vi "Find_camera.vi"(0 "error in":errorcluster) -> (4 "attribs":variant, 5 "port":u16, 6 "error out":errorcluster, 7 "name":string, 8 "CameraInfo":T1 {"serial" format="%x"}, 9 "CameraBase out":refnum<class "CameraBase.lvclass">)   [LabVIEW 2010]
uses:
  <userlib>/Imaging/classes/CameraBase/CameraBase.lvclass
  <userlib>/Imaging/classes/CameraBase/CameraInfo.ctl
  <userlib>/Imaging/classes/sdk_list.ctl
  <userlib>/Imaging/classes/IMAQdx/IMAQdx.lvclass
  <userlib>/Imaging/classes/AndorSDK2/AndorSDK2.lvclass
  <userlib>/h5labview/H5File.lvlib
  <userlib>/h5labview/H5Attrib.lvlib
panel:
  out "h5":path
  in  "cancel":bool
  in  "ok":bool
  in  "cameras":i32(listbox)
  # "Select camera to connect to:"
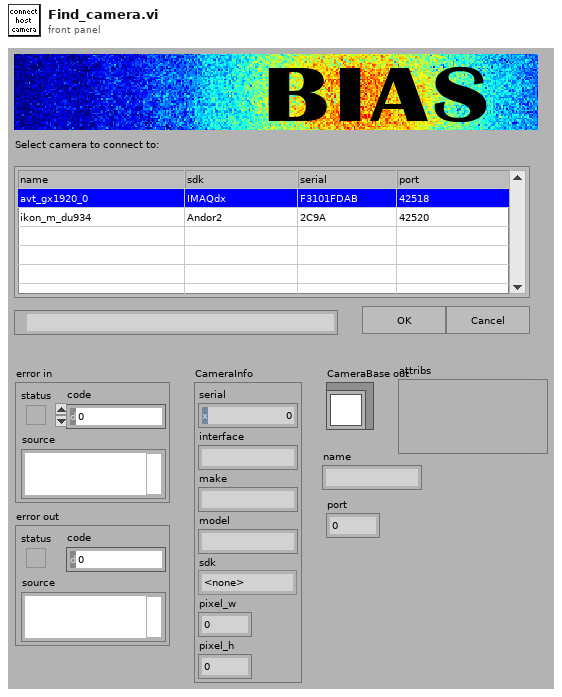
[diagram p1: front panel]
types:
  T1 = typedef "CameraInfo.ctl" = cluster{"serial":u64, "interface":string, "make":string, "model":string, "sdk":T2, "pixel_w":dbl, "pixel_h":dbl}
  T2 = typedef "sdk_list.ctl" = enum16{"<none>", "NIvision", "Andor2", "Andor3"}
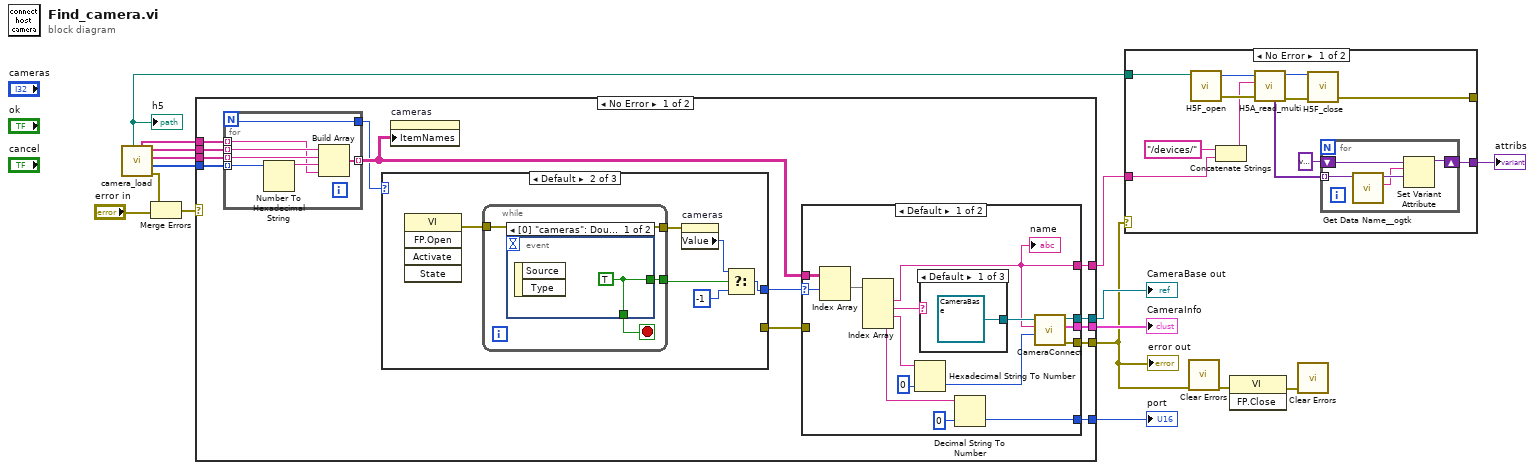
[diagram p0: block diagram]
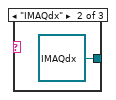
[diagram p3: hidden frame]
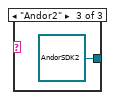
[diagram p4: hidden frame]
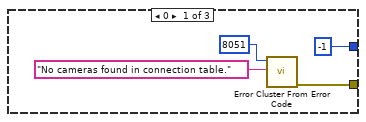
[diagram p6: hidden frame]
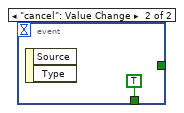
[diagram p7: hidden frame]
diagram:
  n1 = call <userlib>:"camera_load.vi"() -> ("error out"=w14:errorcluster, "serials"=w11:u64[], "sdks"=w10:string[], "names"=w9:string[], "ports"=w8:string[], "hdf"=w5:path)  [unwired: 4 in]
  "h5" <- w5
  n2 = Merge Errors(w14, "error in") -> (w12:errorcluster)
  n3 = case shown="No Error" w12 {
    selector: w12 -> [_ w71]
    tunnel: [w27 w71] -> w2
    tunnel: [w26 _] -> w16
    tunnel: [w25 _] -> w15
    tunnel: w11 -> [w24 _]
    tunnel: w10 -> [w23 _]
    tunnel: w9 -> [w22 _]
    tunnel: w8 -> [w21 _]
    tunnel: [w19 _] -> w7
    tunnel: [w17 _] -> w4
    frame No Error {
      n4 = for {
        N -> [w30]
        tunnel: w22 -> [w36] mode=indexing
        tunnel: w23 -> [w35] mode=indexing
        tunnel: w24 -> [w34] mode=indexing
        tunnel: [w32] -> w20 mode=indexing
        tunnel: w21 -> [w31] mode=indexing
        tunnel: [w30] -> w18
        n5 = Number To Hexadecimal String(2:w34) -> (0:w33:string)  [unwired: 1 in]
        n6 = Build Array(w36, w35, w33, w31) -> (w32:string[])
      }
      n7 = case shown="Default" w18 {
        tunnel: [w58 _ _] -> w28
        tunnel: [-1 ("Value") w61 _] -> w29
        frame 0 {
          n8 = call <vilib>:"Error Cluster From Error Code.vi"("error message (\"\")"="No cameras found in connection table." ("format string"), "error code (0)"=8051) -> ("error out"=w58:errorcluster)  [unwired: 7 in]
        }
        frame Default {
          n9 = invoke class="VI" method="FP.Open"() -> (error out=w60:errorcluster)  [unwired: 5 in, 4 out]
          n10 = while {
            tunnel: w60 -> [w67]
            tunnel: [w68] -> w63
            tunnel: [w67] -> w65
            stop <- w66 stop-if-true
            n11 = event shown="[0] \"cameras\": Double Click;  \"ok\": Value Change" {
              selector: _ -> [_ _]
              dyn-events: _ -> [_ _]
              timeout: _ -> [_ _]
              tunnel: [w69 _] -> w68
              tunnel: [w69 TRUE ("ok")] -> w66
              event "cameras": Double Click; "ok": Value Change {
                w69 = TRUE ("ok")
                n12 = event-data() -> ()  [unwired: 1 in, 2 out]
              }
              event "cancel": Value Change {
                n13 = event-data() -> ()  [unwired: 1 in, 2 out]
              }
            }
          }
          n14 = property on="cameras" class="MCListbox (strict)"(error in=w65) -> ("Value"=w64:i32)  [unwired: 1 in, 2 out]
          n15 = Select(t=w64, s=w63, f=-1) -> (s? t:f=w61:i32)
        }
        frame 1 {
        }
      }
      n16 = property on="cameras" class="MCListbox (strict)"("ItemNames"=w20) -> ()  [unwired: 2 in, 2 out]
      n17 = case shown="Default" w29 {
        selector: w29 -> [w51 _]
        tunnel: w28 -> [_ w55]
        tunnel: w20 -> [w50 _]
        tunnel: [w46 w55] -> w27
        tunnel: [w45 _] -> w26
        tunnel: [w44 _] -> w25
        tunnel: [w37 _] -> w17
        tunnel: [w41 _] -> w19
        frame Default {
          n18 = Index Array(array=w50, index (row)=w51) -> (element=w43:string[])  [unwired: 1 in]
          n19 = Index Array(array=w43) -> (element #1=w37:string, element #2=w40:string, element #3=w39:string, element #4=w42:string)  [unwired: 4 in]
          "name" <- w37
          n20 = Hexadecimal String To Number(string=w39, default (0uL)=u64 0 ("default (0 U32)")) -> (number=w47:u64)  [unwired: 1 in, 1 out]
          n21 = case shown="Default" w40 {
            tunnel: [refnum<class "CameraBase.lvclass"> refnum ("CameraBase.lvclass") refnum<class "IMAQdx.lvclass"> refnum ("IMAQdx.lvclass") refnum<class "AndorSDK2.lvclass"> refnum ("AndorSDK2.lvclass")] -> w49
            frame Default {
            }
            frame "IMAQdx" {
            }
            frame "Andor2" {
            }
          }
          n22 = Decimal String To Number(string=w42, default (0L)=u16 0 ("default (0 I32)")) -> (number=w41:u16)  [unwired: 1 in, 1 out]
          n23 = call-dynamic "CameraConnect.vi"("serial"=w47, "name"=w37, "CameraBase in"=w49) -> ("error out"=w46:errorcluster, "CameraInfo"=w45:T1, "CameraBase out"=w44:refnum<class "CameraBase.lvclass">)  [unwired: 6 in]
        }
        frame -1 {
        }
      }
    }
    frame Error {
    }
  }
  "CameraBase out" <- w15
  "error out" <- w2
  "CameraInfo" <- w16
  "port" <- w7
  n24 = case shown="No Error" w2 {
    tunnel: w5 -> [w83 _]
    tunnel: w4 -> [w81 _]
    tunnel: [w73 _] -> w3
    tunnel: [w72 _] -> _
    frame No Error {
      n25 = call <userlib>:"H5F_open.vi"("path"=w83) -> ("error out"=w78:errorcluster, "ref"=w80:i32)  [unwired: 3 in]
      n26 = Concatenate Strings("/devices/", w81) -> (w76:string)
      n27 = call <userlib>:"H5A_read_multi.vi"("error in (no error)"=w78, "obj_name"=w76, "ref"=w80) -> ("error out"=w77:errorcluster, "ref out"=w79:i32, "attribs"=w75:variant[])  [unwired: 4 in]
      n28 = call <userlib>:"H5F_close.vi"("error in (no error)"=w77, "ref"=w79) -> ("error out"=w72:errorcluster)  [unwired: 3 in]
      n29 = for {
        tunnel: w75 -> [w86] mode=indexing
        shift-right: [w85] -> w73
        shift-left: variant ("variant") -> [w84]
        n30 = call <userlib>:"Get Data Name__ogtk.vi"("Data"=w86) -> ("Data Name"=w87:string, "Data dup"=w88:variant)  [unwired: 8 in, 1 out]
        n31 = Set Variant Attribute(Variant=w84, name=w87, value=w88) -> (Variant out=w85:variant)  [unwired: 1 in, 2 out]
      }
    }
    frame Error {
    }
  }
  "attribs" <- w3
  n32 = call <vilib>:"Clear Errors.vi"("error in (no error)"=w2) -> ("error out"=w6:errorcluster)  [unwired: 6 in]
  n33 = invoke class="VI" method="FP.Close"(error in=w6) -> (error out=w1:errorcluster)  [unwired: 2 in, 2 out]
  n34 = call <vilib>:"Clear Errors.vi"("error in (no error)"=w1) -> ()  [unwired: 6 in, 1 out]
